vi "Graph_legend (SubVI).vi"(6 "Numeric":i32, 7 "rb":i32, 9 "String":string, 11 "appended array":refnum<vi>[](array[refnum])) -> ()   [LabVIEW 2017]
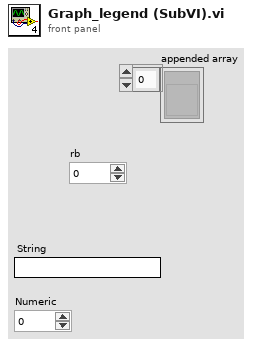
[diagram p1: front panel]
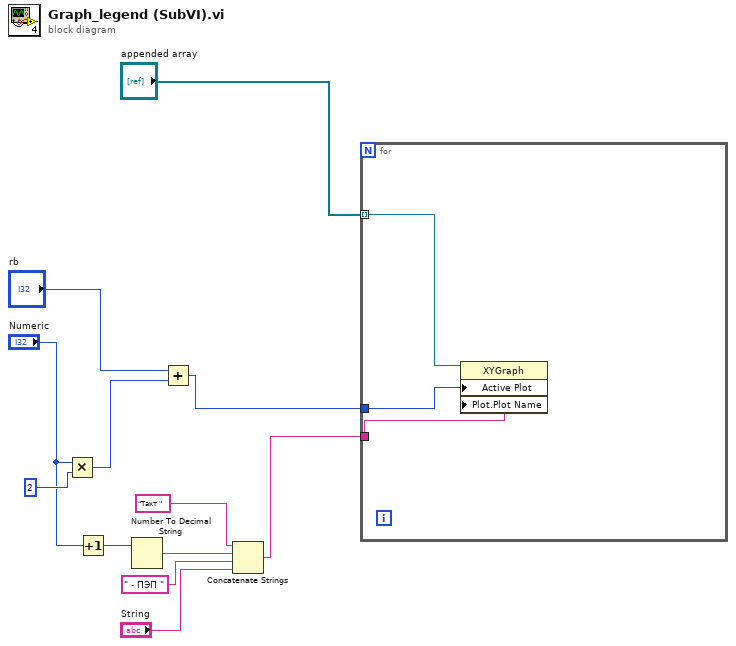
[diagram p0: block diagram]
diagram:
  n1 = Multiply(x="Numeric", y=2) -> (x*y=w7:i32)
  n2 = Increment(x="Numeric") -> (x+1=w4:i32)
  n3 = Number To Decimal String(number=w4) -> (decimal integer string=w9:string)  [unwired: 1 in]
  n4 = Add(x="rb", y=w7) -> (x+y=w3:i32)
  n5 = Concatenate Strings("Такт " ("string"), w9, " - ПЭП " ("string"), "String") -> (w2:string)
  n6 = for {
    tunnel: "appended array" -> [w13] mode=indexing
    tunnel: w3 -> [w15]
    tunnel: w2 -> [w14]
    n7 = property on="Property Node" class="XYGraph"(reference=w13, "Active Plot"=w15, "Plot.Plot Name"=w14) -> ()  [unwired: 1 in, 2 out]
  }
